vi "Log CSV.vi"() -> ()   [LabVIEW 2024]
uses:
  controls/GlobalData.ctl
  <vilib>/Utility/config.llb/NI_LVConfig.lvlib
panel:
  in  "error in (no error)":errorcluster
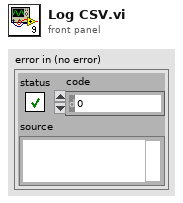
[diagram p1: front panel]
types:
  T1 = typedef "GlobalData.ctl" = cluster{"Measurements":cluster{"Measurement Graphs":refnum<vi>, "Pressure":refnum<vi>, "Temperature":refnum<vi>, "Salinity":refnum<vi>, "Weight":refnum<vi>, "Pressure Raw":refnum<vi>, "Temperature Raw":refnum<vi>, "Salinity Raw":refnum<vi>, "Weight Raw":refnum<vi>, "Measurement Statstics":refnum<vi>, "Time Array":refnum<vi>}, "Settings":cluster{"Sampling Settings":refnum<vi>, "General Settings":refnum<vi>, "Disable Sensor Reading":refnum<vi>, "Units Settings":refnum<vi>, "Channels Settings":refnum<vi>, "Weight Port Settings":refnum<vi>}, "Calibration Data":cluster{"Pressure Cal":refnum<vi>, "Temperature Cal":refnum<vi>, "Salinity Cal":refnum<vi>, "Weight Cal":refnum<vi>}, "UI":cluster{"Generate Report":refnum<vi>}}
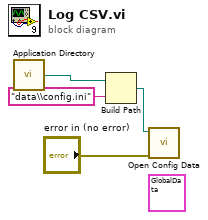
[diagram p0: block diagram]
diagram:
  (unwired) T1 {"Measurements"={"Measurement Graphs"=refnum, "Pressure"=refnum, "Temperature"=refnum, "Salinity"=refnum, "Weight"=refnum, "Pressure Raw"=refnum, "Temperature Raw"=refnum, "Salinity Raw"=refnum, "Weight Raw"=refnum, "Measurement Statstics"=refnum, "Time Array"=refnum}, "Settings"={"Sampling Settings"=refnum, "General Settings"=refnum, "Disable Sensor Reading"=refnum, "Units Settings"=refnum, "Channels Settings"=refnum, "Weight Port Settings"=refnum}, "Calibration Data"={"Pressure Cal"=refnum, "Temperature Cal"=refnum, "Salinity Cal"=refnum, "Weight Cal"=refnum}, "UI"={"Generate Report"=refnum}} ("GlobalData")
  n1 = call <vilib>:"Application Directory.vi"() -> ("Application Directory"=w1:path)
  n2 = Build Path(base path=w1, name or relative path="data\\config.ini") -> (appended path=w2:path)
  n3 = call <vilib>:"Open Config Data.vi"("error in (no error)"="error in (no error)", "configuration file path"=w2) -> ()  [unwired: 7 in, 3 out]
